vi "GrapFramesRollingBuffer.vi"(0 "object in":refnum<class "Hamamatsu.lvclass">, 5 "error in (no error)":errorcluster) -> (14 "object out":refnum<class "Hamamatsu.lvclass">, 19 "error out":errorcluster)   [LabVIEW 2021, in "Hamamatsu.lvclass"]
uses:
  Hamamatsu.lvclass
  Hamamatsu.lvclass/Hamamatsu.ctl
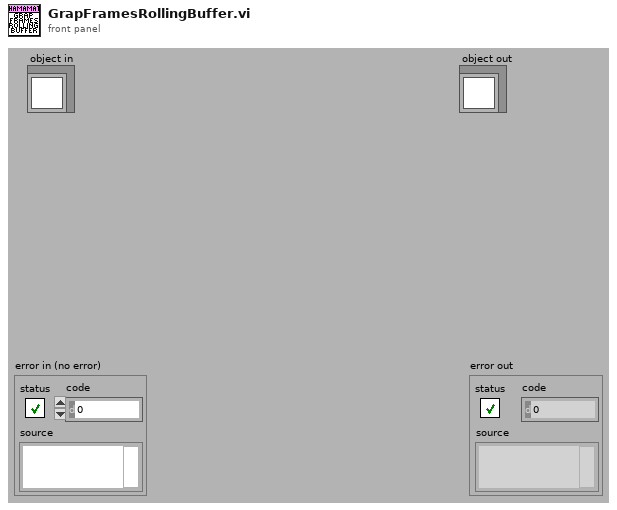
[diagram p1: front panel]
types:
  T1 = typedef "IMAQ Image.ctl" = refnum<image>
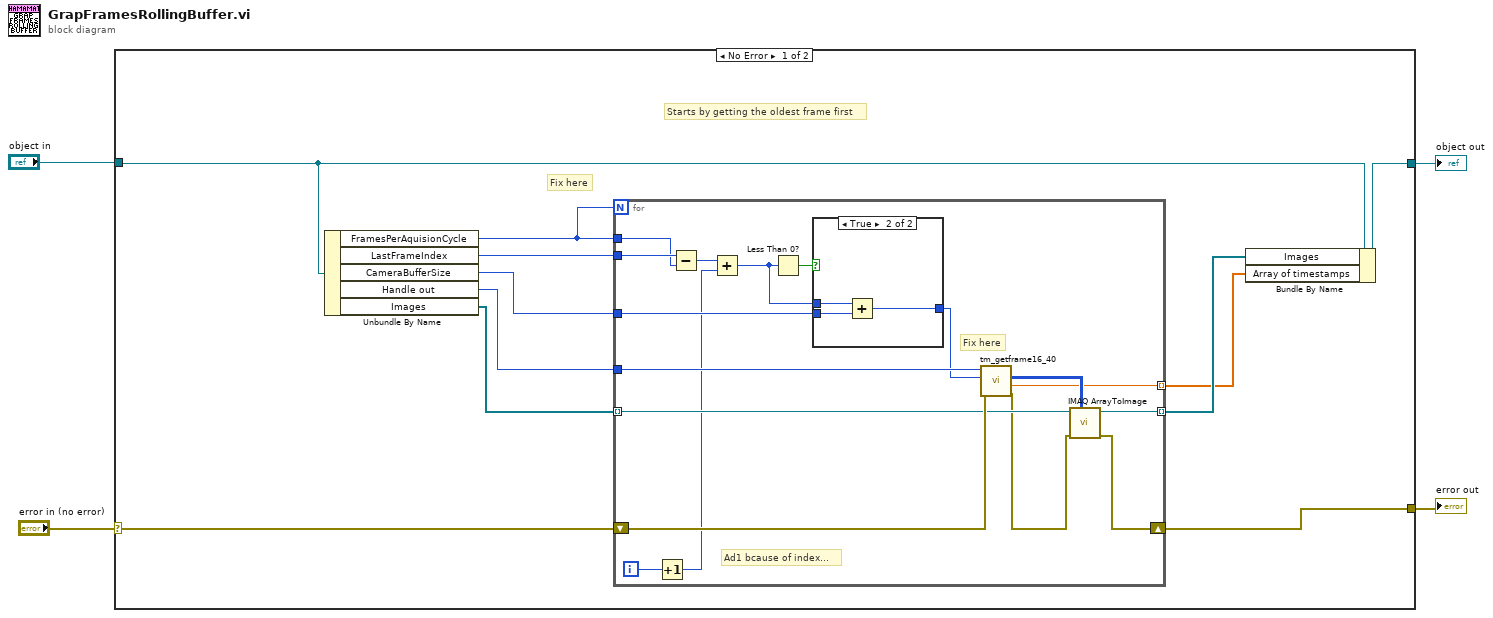
[diagram p0: block diagram]
diagram:
  n1 = case shown="No Error" "error in (no error)" {
    selector: "error in (no error)" -> [w14 w38]
    tunnel: [w13 w38] -> w3
    tunnel: [w15 w37] -> w1
    tunnel: "object in" -> [w12 w37]
    frame No Error {
      # "Starts by getting the oldest frame first"
      # "Fix here"
      n2 = Unbundle By Name(w12) -> ("FramesPerAquisionCycle"=w6:i32, "LastFrameIndex"=w10:i32, "CameraBufferSize"=w9:i32, "Handle out"=w8:u32, "Images"=w7:T1[])
      n3 = for {
        N: w6 -> [_]
        shift-right: [w25] -> w13
        shift-left: w14 -> [w32]
        tunnel: w10 -> [w21]
        tunnel: w6 -> [w19]
        tunnel: w9 -> [w31]
        tunnel: w8 -> [w29]
        tunnel: w7 -> [w27] mode=indexing
        tunnel: [w24] -> w11 mode=indexing
        tunnel: [w16] -> w5 mode=indexing
        i -> [w18]
        # "Ad1 bcause of index..."
        # "Fix here"
        n4 = Increment(x=w18) -> (x+1=w17:i32)
        n5 = Subtract(x=w21, y=w19) -> (x-y=w23:i32)
        n6 = Add(x=w23, y=w17) -> (x+y=w22:i32)
        n7 = Less Than 0?(x=w22) -> (x < 0?=w30:bool)
        n8 = case shown="True" w30 {
          tunnel: w31 -> [_ w36]
          tunnel: w22 -> [w33 w35]
          tunnel: [w33 w34] -> w20
          frame False {
          }
          frame True {
            n9 = Add(x=w35, y=w36) -> (x+y=w34:i32)
          }
        }
        n10 = call <userlib>:"tm_getframe16_40.vi"("error in (no error)"=w32, "Frame Index"=w20, "Handle in"=w29) -> ("error out"=w26:errorcluster, "Timestamp"=w16:dbl, "Data"=w28:u16[][])  [unwired: 5 in, 1 out]
        n11 = call "IMAQ ArrayToImage"("Image Pixels (U16)"=w28, "error in (no error)"=w26, "Image"=w27) -> ("error out"=w25:errorcluster, "Image Out"=w24:T1)  [unwired: 7 in]
      }
      n12 = Bundle By Name(cluster=w12, "Images"=w11, "Array of timestamps"=w5) -> (w15:refnum<class "Hamamatsu.lvclass">)
    }
    frame Error {
    }
  }
  "error out" <- w3
  "object out" <- w1
